vi "destroy.vi"(8 "error in":errorcluster, 11 "results reporter in":refnum<class "results reporter.lvclass">) -> (0 "error out":errorcluster)   [LabVIEW 2013, in "results reporter.lvclass"]
uses:
  results reporter.lvclass
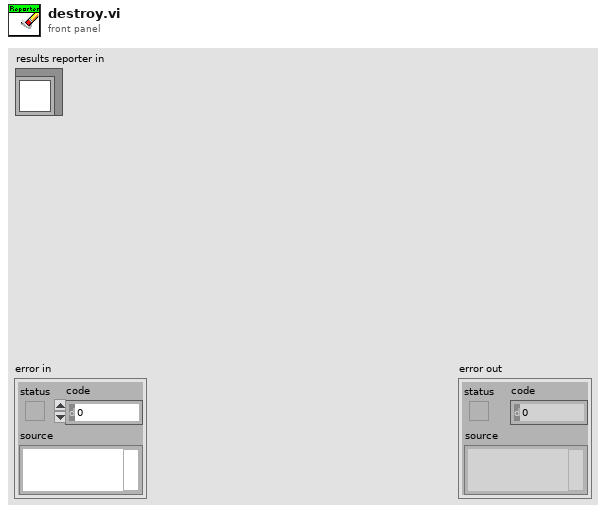
[diagram p1: front panel]
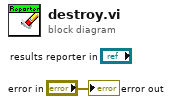
[diagram p0: block diagram]
diagram:
  "error out" <- "error in"
